vi "Check Path.vi"(2 "error in (no error)":errorcluster, 3 "path in":path) -> (0 "error out":errorcluster, 1 "path out":path)   [LabVIEW 2019]
doc: "Checks the path to see if it actually exists on disk. If it does not the error cluster is set. If the path is a relative path, an absolute path is made from the relative path by appending it with the path to the directory in which the top most VI of this program exists."
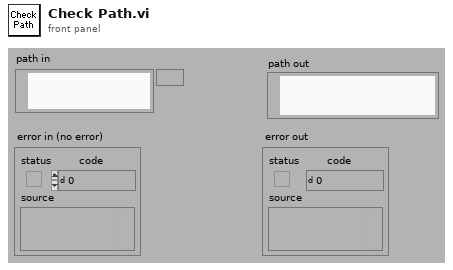
[diagram p1: front panel]
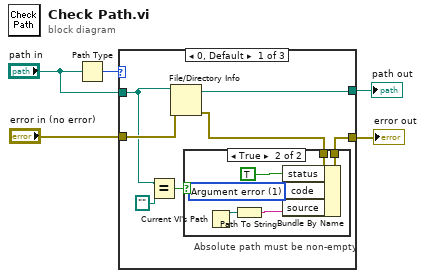
[diagram p0: block diagram]
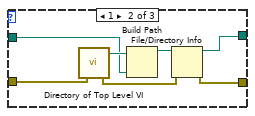
[diagram p3: hidden frame]
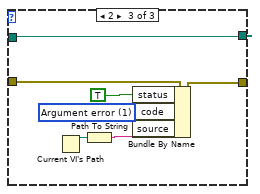
[diagram p4: hidden frame]
diagram:
  n1 = Path Type(1:"path in") -> (0:w5:i16)
  n2 = case shown="0, Default" w5 {
    tunnel: "error in (no error)" -> [w12 w26 w29]
    tunnel: [w9 w21 w28] -> w3
    tunnel: "path in" -> [w6 w24 w27]
    tunnel: [w11 w20 w27] -> w1
    frame 0, Default {
      # "Absolute path must be non-empty"
      n3 = Equal?(x=w6, y=path "") -> (x = y?=w7:bool)
      n4 = File/Directory Info(path=w6, error in=w12) -> (path out=w11:path, error out=w10:errorcluster)  [unwired: 5 out]
      n5 = case shown="True" w7 {
        tunnel: w10 -> [w13 w15]
        tunnel: [w13 w14] -> w9
        frame False {
        }
        frame True {
          w17 = 1 items=["No error", "Argument error", "Memory is full", "Out of zone", "End of file", "File already open", "Generic file I/O error", "File not found", "File permission error", "Disk is full", "Duplicate path", "Too many files open", "System feature not enabled", "Resource file not found", "Cannot add resource", "Resource not found", "Image not found", "Image memory error", "Pen does not exist", "Config type invalid", "Config token not found", "Config parse error", "Config memory error", "Bad external code format", "Bad external code offset", "External code not present", "Null window", "Destroy window error", "Null menu", "Print aborted", "Bad print record", "Print driver error", "Windows error during printing", "Memory error during printing", "Print dialog error", "Generic print error", "Invalid device refnum", "Device not found", "Device parameter error", "Device unit error", "Cannot open device", "Device call aborted", "Generic error", "Cancelled by user", "Object ID too low", "Object ID too high", "Object not in heap", "Unknown heap", "Unknown object (invalid DefProc)", "Unknown object (DefProc not in table)", "Message out of range", "Invalid (null) method", "Unknown message", "Manager call not supported", "Bad address", "Network operation in progress", "Network operation timed out", "Connection is busy", "Network attribute not supported", "Network error", "Address in use", "System out of memory", "Connection aborted", "Connection refused", "Not connected", "Already connected", "Connection closed", "Initialization error (interapplication manager)", "Bad occurrence", "Wait on unbound occurrence handler", "Occurrence queue overflow", "Datalog type conflict", "Unused", "Unrecognized type (interapplication manager)", "Memory corrupt", "Failed to make temporary DLL", "Old CIN version", "Drag socket not found", "Failed to load drop-object", "Failed to register OLE object", "Failed to release OLE object", "Format specifier type mismatch", "Unknown format specifier", "Too few format specifiers", "Too many format specifiers", "Scan failed", "Newer CIN version", "Error converting to variant", "Runtime menu error", "Password tampered", "Variant attribute not found", "Incompatible variant data type", "Event data is not available", "Event Store is not present", "Occurrence is not found", "Event Queue is not created", "Event info is not available", "Refnum passed is NULL", "Error retrieving Class GUID", "Error retrieving CoClass GUID", "Error retrieving TypeLib GUID.", "Bad built application magic bytes.", "Specific driver is different from the specific driver associated with the Logical Name.", "There is no session opened to the class driver.", "Max Error", "MAX - Error with config objects", "MAX - Error loading configuration", "MAX - Group not supported"]
          n6 = Current VI's Path() -> (path=w18:path)
          n7 = Path To String(path=w18) -> (string=w19:string)
          n8 = Bundle By Name(cluster=w15, "status"=TRUE, "code"=w17, "source"=w19) -> (w14:errorcluster)
        }
      }
    }
    frame 1 {
      n9 = call "Directory of Top Level VI.vi"("error in (no error)"=w26) -> ("directory of top VI"=w25:path, "error out"=w22:errorcluster)
      n10 = Build Path(base path=w25, name or relative path=w24) -> (appended path=w23:path)
      n11 = File/Directory Info(path=w23, error in=w22) -> (path out=w20:path, error out=w21:errorcluster)  [unwired: 5 out]
    }
    frame 2 {
      w31 = 1 items=["No error", "Argument error", "Memory is full", "Out of zone", "End of file", "File already open", "Generic file I/O error", "File not found", "File permission error", "Disk is full", "Duplicate path", "Too many files open", "System feature not enabled", "Resource file not found", "Cannot add resource", "Resource not found", "Image not found", "Image memory error", "Pen does not exist", "Config type invalid", "Config token not found", "Config parse error", "Config memory error", "Bad external code format", "Bad external code offset", "External code not present", "Null window", "Destroy window error", "Null menu", "Print aborted", "Bad print record", "Print driver error", "Windows error during printing", "Memory error during printing", "Print dialog error", "Generic print error", "Invalid device refnum", "Device not found", "Device parameter error", "Device unit error", "Cannot open device", "Device call aborted", "Generic error", "Cancelled by user", "Object ID too low", "Object ID too high", "Object not in heap", "Unknown heap", "Unknown object (invalid DefProc)", "Unknown object (DefProc not in table)", "Message out of range", "Invalid (null) method", "Unknown message", "Manager call not supported", "Bad address", "Network operation in progress", "Network operation timed out", "Connection is busy", "Network attribute not supported", "Network error", "Address in use", "System out of memory", "Connection aborted", "Connection refused", "Not connected", "Already connected", "Connection closed", "Initialization error (interapplication manager)", "Bad occurrence", "Wait on unbound occurrence handler", "Occurrence queue overflow", "Datalog type conflict", "Unused", "Unrecognized type (interapplication manager)", "Memory corrupt", "Failed to make temporary DLL", "Old CIN version", "Drag socket not found", "Failed to load drop-object", "Failed to register OLE object", "Failed to release OLE object", "Format specifier type mismatch", "Unknown format specifier", "Too few format specifiers", "Too many format specifiers", "Scan failed", "Newer CIN version", "Error converting to variant", "Runtime menu error", "Password tampered", "Variant attribute not found", "Incompatible variant data type", "Event data is not available", "Event Store is not present", "Occurrence is not found", "Event Queue is not created", "Event info is not available", "Refnum passed is NULL", "Error retrieving Class GUID", "Error retrieving CoClass GUID", "Error retrieving TypeLib GUID.", "Bad built application magic bytes.", "Specific driver is different from the specific driver associated with the Logical Name.", "There is no session opened to the class driver.", "Max Error", "MAX - Error with config objects", "MAX - Error loading configuration", "MAX - Group not supported"]
      n12 = Current VI's Path() -> (path=w32:path)
      n13 = Path To String(path=w32) -> (string=w33:string)
      n14 = Bundle By Name(cluster=w29, "status"=TRUE, "code"=w31, "source"=w33) -> (w28:errorcluster)
    }
  }
  "error out" <- w3
  "path out" <- w1
